vi "wmlf Example Script.vi"(8 "error in (no error)":errorcluster, 11 "c2dArray":dbl[][](array[numeric])) -> (0 "error out":errorcluster, 2 "function return":i32, 3 "c2dArray out":dbl[][](array[numeric]))   [LabVIEW 2014, in "exampleWrapper.lvlib"]
doc: "int wmlfExampleScript(double* c2dArray, int numRows, int numColumns);"
uses:
  exampleWrapper.lvlib
  <userlib>/exampleWrapper/exampleWrapper.dll
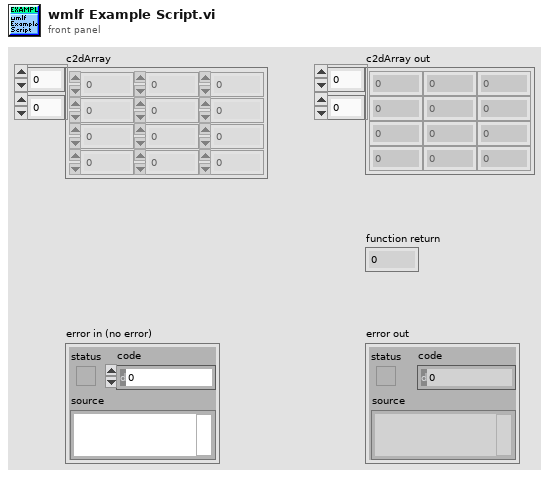
[diagram p1: front panel]
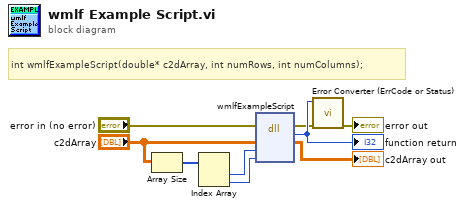
[diagram p0: block diagram]
diagram:
  # "int wmlfExampleScript(double* c2dArray, int numRows, int numColumns);"
  n1 = Array Size(array="c2dArray") -> (size(s)=w3:i32[])
  n2 = Index Array(array=w3) -> (element #1=w2:i32, element #2=w1:i32)  [unwired: 2 in]
  n3 = dll-call lib="C:/Program Files/National Instruments/LabVIEW 2018/user.lib/exampleWrapper/exampleWrapper.*" fn="wmlfExampleScript"(error in="error in (no error)", "c2dArray"="c2dArray", "numRows"=w2, "numColumns"=w1) -> (error out=w6:errorcluster, "return type"=w9:i32, "c2dArray"=→"c2dArray out":dbl[][])  [unwired: 4 in, 1 out]
  "function return" <- w9
  n4 = call "Error Converter (ErrCode or Status).vi"("error in (no error)"=w6, "error code"=w9) -> ("error out"=→"error out":errorcluster)  [unwired: 9 in]
